vi "Periodic Tasks.vi"(8 "error in":errorcluster) -> ()   [LabVIEW 2014]
doc: "This VI runs in parallel to other tasks. It can contain as many user-defined periodic loops as you need. These can carry out PID or other sorts of timed response."
uses:
  <vilib>/Rock Robotics/WPI/Camera/WPI_CameraImageSize.ctl
  <vilib>/Rock Robotics/WPI/Camera/WPI_CameraFrameRate.ctl
  <vilib>/Rock Robotics/WPI/Joystick/WPI_JoystickGetSetRefNum.vi
  <vilib>/Rock Robotics/WPI/RobotDrive/WPI_RobotDriveGetSetRefNum.vi
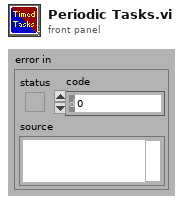
[diagram p1: front panel]
types:
  T1 = typedef "Image Type" = u32
  T2 = typedef "WPI_CameraFrameRate.ctl" = u32
  T3 = typedef "WPI_CameraImageSize.ctl" = enum16{"640x480", "320x240", "160x120", "Custom"}
  T4 = typedef "WPI_JoystickDevRef.ctl" = cluster{"Device":T5}
  T5 = typedef "WPI_JoystickDeviceEnum.ctl" = enum16{"USB 0", "USB 1", "USB 2", "USB 3", "USB 4", "USB 5"}
  T6 = typedef "WPI_RobotDriveDevRef.ctl" = cluster{"DevStatus":errorcluster, "Motors[]":T7[], "Square Inputs":bool, "Max Output":dbl}
  T7 = typedef "WPI_MotorControlDeviceRef.ctl" = cluster{"DeviceStatus":errorcluster, "Type":T8, "PWM":cluster{"Controller":T9, "PWM Channel":T10, "DeadBand":T11}, "CAN":cluster{"Device Number":u8, "Control Mode":T12, "Semaphore":T13, "Max Vout":dbl, "TalonSRX Control Mode":T14}, "Invert":bool, "TransformRef":T15, "InvTransformRef":T15}
  T8 = typedef "WPI_MotorControlType.ctl" = enum16{"PWM", "CAN", "CANTalonSRX"}
  T9 = typedef "FPGA_TypedefDigitalModule.ctl" = enum16{"Controller 1"}
  T10 = typedef "FPGA_DIOPWMChannel.ctl" = enum8{"PWM 0", "PWM 1", "PWM 2", "PWM 3", "PWM 4", "PWM 5", "PWM 6", "PWM 7", "PWM 8", "PWM 9", "PWM MXP 0", "PWM MXP 1", "PWM MXP 2", "PWM MXP 3", "PWM MXP 4", "PWM MXP 5", "PWM MXP 6", "PWM MXP 7", "PWM MXP 8", "PWM MXP 9", "Invalid"}
  T11 = typedef "WPI_PWMDeadband.ctl" = cluster{"Name":string, "maxPositivePwm":i32, "minPositivePwm":i32, "centerPwm":i32, "maxNegativePwm":i32, "minNegativePwm":i32, "angularRange":u16}
  T12 = typedef "WPI_CANJaguar_ControlMode.ctl" = enum8{"Percent VBus", "Current", "Speed", "Position", "Voltage"}
  T13 = typedef "Semaphore RefNum" = refnum<k1>
  T14 = typedef "WPI_CANTalonSRX_APIControlMode.ctl" = enum8{"Percent VBus", "Speed", "Position", "Slave", "Unchanged / Invalid"}
  T15 = typedef "WPI_PWMTransform_ConPane.ctl" = refnum<vi>
  T16 = typedef "WPI_CameraDevRef.ctl" = cluster{"Camera Address":string, "CameraStatus":errorcluster}
  T17 = cluster{"JoystickDevRef":T4, "RobotDriveDevRef":T6}
  T18 = typedef "IMAQ Image.ctl" = refnum<image>
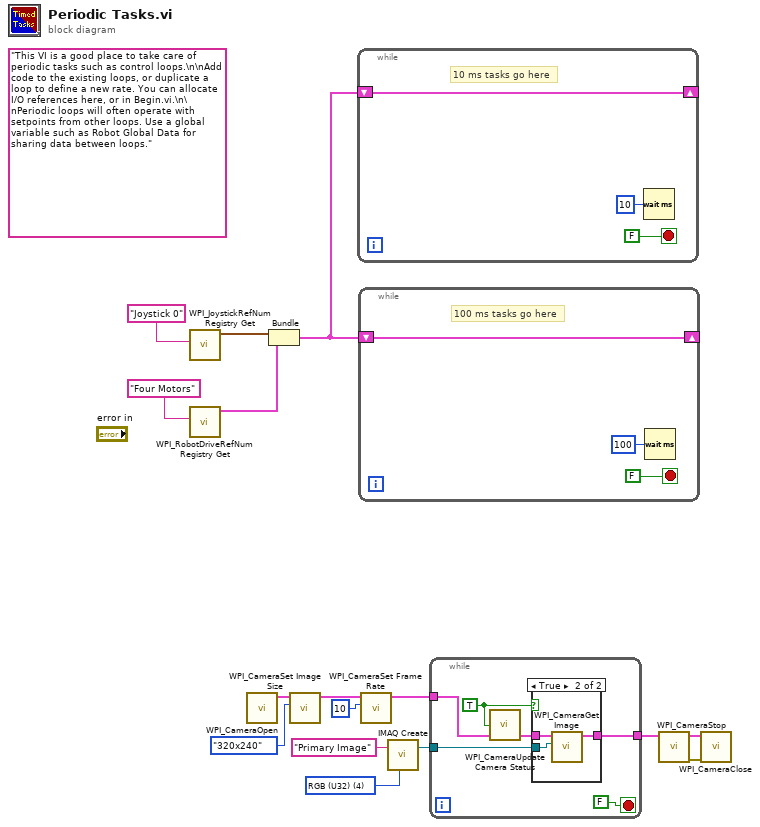
[diagram p0: block diagram]
diagram:
  w1 = T1 4 items=["Grayscale (U8)", "Grayscale (I16)", "Grayscale (SGL)", "Complex (CSG)", "RGB (U32)", "HSL (U32)", "RGB (U64)", "Grayscale (U16)"] ("Image Type")
  (unwired) "This VI is a good place to take care of periodic tasks such as control loops.\n\nAdd code to the existing loops, or duplicate a loop to define a new rate. You can allocate I/O references here, or in Begin.vi.\n\nPeriodic loops will often operate with setpoints from other loops. Use a global variable such as Robot Global Data for sharing data between loops."
  n1 = call <vilib>:"WPI_JoystickRefNum Registry Get.vi"("refnum name"="Joystick 0") -> ("JoystickDevRef"=w14:T4)  [unwired: 1 in, 9 out]
  n2 = call <vilib>:"WPI_RobotDriveRefNum Registry Get.vi"("refnum name"="Four Motors") -> ("RobotDriveDevRef"=w13:T6)  [unwired: 1 in, 9 out]
  n3 = call <vilib>:"WPI_CameraOpen.vi"() -> ("CameraDevRef"=w10:T16)  [unwired: 10 in, 1 out]
  n4 = Bundle("JoystickDevRef"=w14, "RobotDriveDevRef"=w13) -> (w12:T17)  [unwired: 1 out]
  n5 = call <vilib>:"WPI_CameraSet Image Size.vi"("Image Size"=WPI_CameraImageSize."320x240", "CameraDevRef"=w10) -> ("CameraDevRef Out"=w9:T16)  [unwired: 8 in, 1 out]
  n6 = while {
    shift-right: [w17] -> _
    shift-left: w12 -> [w17]
    stop <- FALSE stop-if-true
    # "10 ms tasks go here"
    n7 = Wait (ms)(milliseconds to wait=u32 10) -> ()  [unwired: 1 out]
  }
  n8 = while {
    shift-right: [w20] -> _
    shift-left: w12 -> [w20]
    stop <- FALSE stop-if-true
    # "100 ms tasks go here"
    n9 = Wait (ms)(milliseconds to wait=u32 100) -> ()  [unwired: 1 out]
  }
  n10 = call <vilib>:"WPI_CameraSet Frame Rate.vi"("Frame Rate (fps)"=T2 10, "CameraDevRef"=w9) -> ("CameraDevRef Out"=w8:T16)  [unwired: 8 in, 1 out]
  n11 = call "IMAQ Create"("Image Name"="Primary Image", "Image Type"=w1) -> ("New Image"=w3:T18)  [unwired: 3 in, 1 out]
  n12 = while {
    tunnel: w8 -> [w28]
    tunnel: [w26] -> w7
    tunnel: w3 -> [w25]
    stop <- FALSE stop-if-true
    w24 = TRUE ("Enable Vision")
    n13 = call <vilib>:"WPI_CameraUpdate Camera Status.vi"("CameraDevRef In"=w28, "Enable Vision"=w24) -> ("CameraDevRef Out"=w27:T16)  [unwired: 3 in]
    n14 = case shown="True" w24 {
      tunnel: w27 -> [w29 w32]
      tunnel: [w29 w31] -> w26
      tunnel: w25 -> [_ w30]
      frame False {
      }
      frame True {
        n15 = call <vilib>:"WPI_CameraGet Image.vi"("Image"=w30, "CameraDevRef"=w32) -> ("CameraDevRef Out"=w31:T16)  [unwired: 7 in, 2 out]
      }
    }
  }
  n16 = call <vilib>:"WPI_CameraStop.vi"("CameraDevRef"=w7) -> ("error out"=w4:errorcluster, "CameraDevRef Out"=w11:T16)  [unwired: 9 in]
  n17 = call <vilib>:"WPI_CameraClose.vi"("error in (no error)"=w4, "CameraDevRef"=w11) -> ()  [unwired: 9 in, 1 out]
